vi "zadanie_1.vi"() -> ()   [LabVIEW 2020]
panel:
  in  "Opoznienie wykonania petli For [ms]":u32
  in  "Zatrzymaj program":bool
  in  "Wprowadz liczbe wykonan petli For":i32
  out "Ilosc wykonan petli For":i32
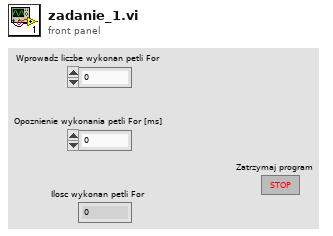
[diagram p1: front panel]
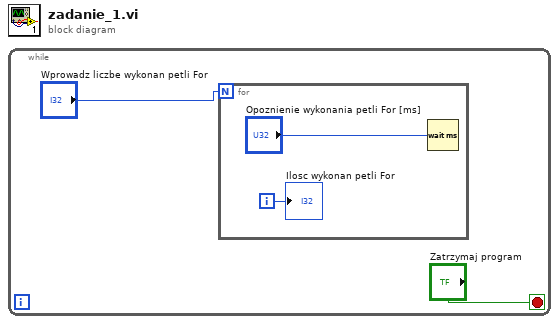
[diagram p0: block diagram]
diagram:
  n1 = while {
    stop <- "Zatrzymaj program" stop-if-true
    n2 = for {
      N: "Wprowadz liczbe wykonan petli For" -> [_]
      i -> [w3]
      n3 = Wait (ms)(milliseconds to wait="Opoznienie wykonania petli For [ms]") -> ()  [unwired: 1 out]
      "Ilosc wykonan petli For" <- w3
    }
  }
